vi "Multistate Facade.vi"(0 "Data In":T3, 2 "Display State In":T2, 3 "Container State":T4) -> (6 "Data Out":T3, 7 "Display State Out":T2, 8 "Action":T1)   [LabVIEW 2019, in "MultiStateLED.xctl"]
uses:
  MultiStateLED.xctl
  Multistate Out Data.ctl
  <vilib>/_xctls/Container State.ctl
  Simple Error Out State.ctl
  <vilib>/_xctls/Action.ctl
  <vilib>/_xctls/XControlSupport.lvlib
panel:
  out "error out":bool=TRUE
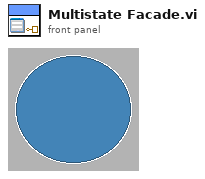
[diagram p1: front panel]
types:
  T1 = typedef "XControlSupport.lvlib/Action.ctl" = cluster{"Data Changed?":bool, "State Changed?":bool, "Action Name":string}
  T2 = typedef "MultiStateLED.xctl/Simple Error Out State.ctl" = cluster{"State":T3}
  T3 = typedef "MultiStateLED.xctl/Multistate Out Data.ctl" = enum16{"Idle", "Green", "Red", "Orange"}
  T4 = typedef "XControlSupport.lvlib/Container State.ctl" = cluster{"Indicator?":bool, "Run Mode?":bool, " Refnum":refnum<vi>}
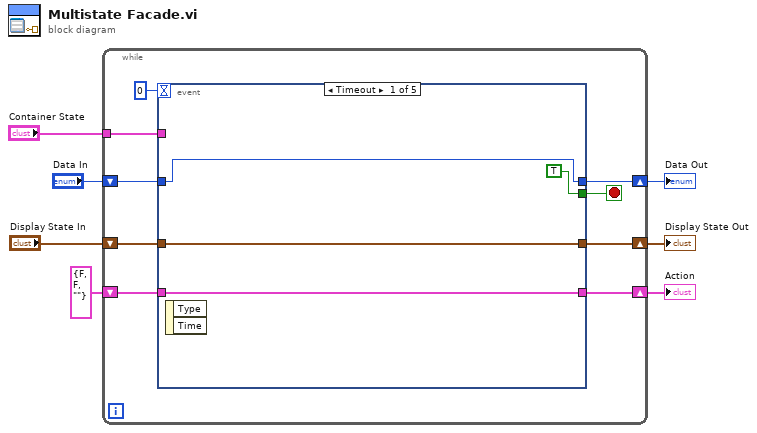
[diagram p0: block diagram]
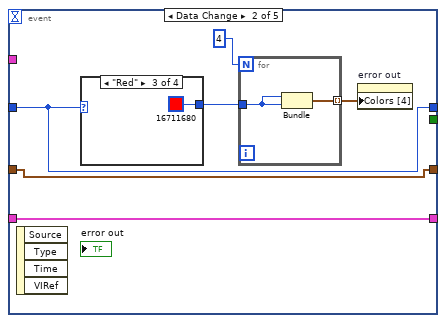
[diagram p2: hidden frame]
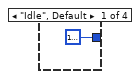
[diagram p3: hidden frame]
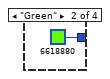
[diagram p4: hidden frame]
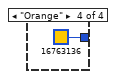
[diagram p5: hidden frame]
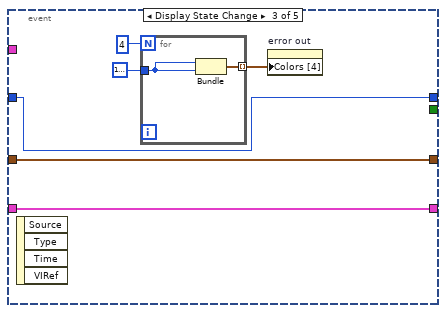
[diagram p6: hidden frame]
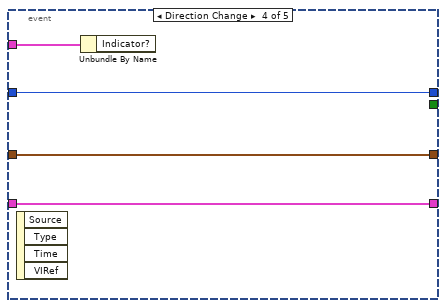
[diagram p7: hidden frame]
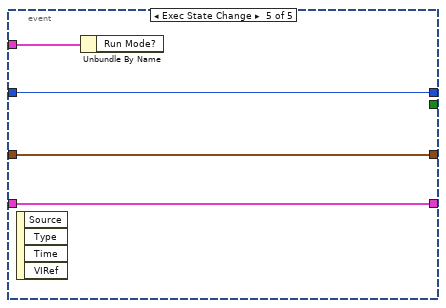
[diagram p8: hidden frame]
diagram:
  n1 = while {
    shift-right: [w15] -> w4
    shift-left: "Display State In" -> [w16]
    tunnel: "Container State" -> [w12]
    shift-right: [w10] -> w7
    shift-left: "Data In" -> [w11]
    shift-right: [w8] -> w2
    shift-left: T1 {"Data Changed?"=FALSE, "State Changed?"=FALSE, "Action Name"=""} ("Action") -> [w9]
    stop <- w14 stop-if-true
    n2 = event shown="[0] Timeout" {
      selector: _ -> [_ _ _ _ _]
      dyn-events: _ -> [_ _ _ _ _]
      timeout: 0 -> [_ _ _ _ _]
      tunnel: w16 -> [w18 w26 w38 w43 w47]
      tunnel: [w18 w26 w38 w43 w47] -> w15
      tunnel: [TRUE _ _ _ _] -> w14
      tunnel: w12 -> [_ _ _ w44 w48]
      tunnel: w11 -> [w17 w22 w37 w42 w46]
      tunnel: [w17 w22 w37 w42 w46] -> w10
      tunnel: [w19 w25 w36 w41 w45] -> w8
      tunnel: w9 -> [w19 w25 w36 w41 w45]
      event Timeout {
        n3 = event-data() -> ()  [unwired: 1 in, 2 out]
      }
      event Data Change {
        n4 = event-data() -> ()  [unwired: 1 in, 4 out]
        n5 = case shown="\"Red\"" w22 {
          tunnel: [u32 16777216 u32 6618880 u32 16711680 u32 16763136] -> w21
          frame "Idle", Default {
          }
          frame "Green" {
          }
          frame "Red" {
          }
          frame "Orange" {
          }
        }
        n6 = for {
          N: 4 -> [_]
          tunnel: w21 -> [w32]
          tunnel: [w31] -> w23 mode=indexing
          n7 = Bundle(w32, w32) -> (w31:cluster{u32, u32})  [unwired: 1 in]
        }
        n8 = property on="error out" class="Bool (strict)"("Colors [4]"=w23) -> ()  [unwired: 2 in, 2 out]
      }
      event Display State Change {
        n9 = event-data() -> ()  [unwired: 1 in, 4 out]
        n10 = for {
          N: 4 -> [_]
          tunnel: u32 16777216 -> [w40]
          tunnel: [w39] -> w34 mode=indexing
          n11 = Bundle(w40, w40) -> (w39:cluster{u32, u32})  [unwired: 1 in]
        }
        n12 = property on="error out" class="Bool (strict)"("Colors [4]"=w34) -> ()  [unwired: 2 in, 2 out]
      }
      event Direction Change {
        n13 = event-data() -> ()  [unwired: 1 in, 4 out]
        n14 = Unbundle By Name(w44) -> ()  [unwired: 1 out]
      }
      event Exec State Change {
        n15 = event-data() -> ()  [unwired: 1 in, 4 out]
        n16 = Unbundle By Name(w48) -> ()  [unwired: 1 out]
      }
    }
  }
  "Display State Out" <- w4
  "Data Out" <- w7
  "Action" <- w2
